vi "Copy of plot states.vi"() -> ()   [LabVIEW 2017]
panel:
  out "Ts Diagram":cluster{dbl[], dbl[]}[](graph)
  out "ph Diagram":cluster{dbl[], dbl[]}[](graph)
  out "Ts Sat Curve":cluster{dbl[], dbl[]}
  out "ph Sat Curve":cluster{dbl[], dbl[]}
  out "Ts output":cluster{dbl[], dbl[]}
  out "ph output":cluster{dbl[], dbl[]}
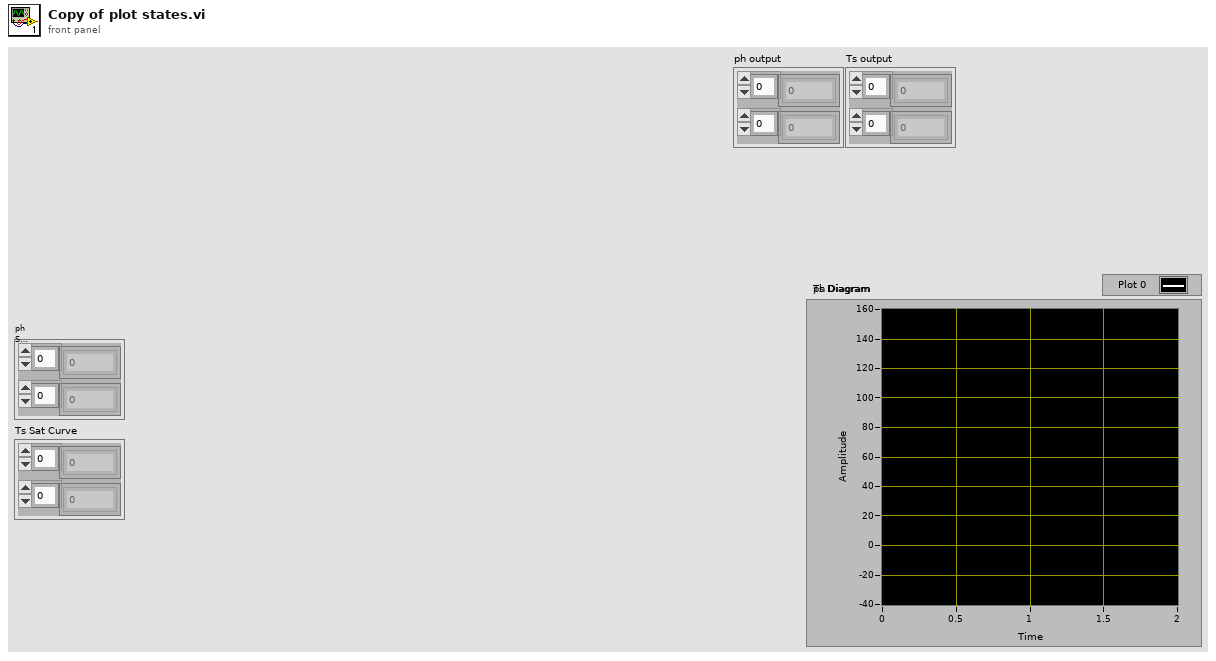
[diagram p1: front panel]
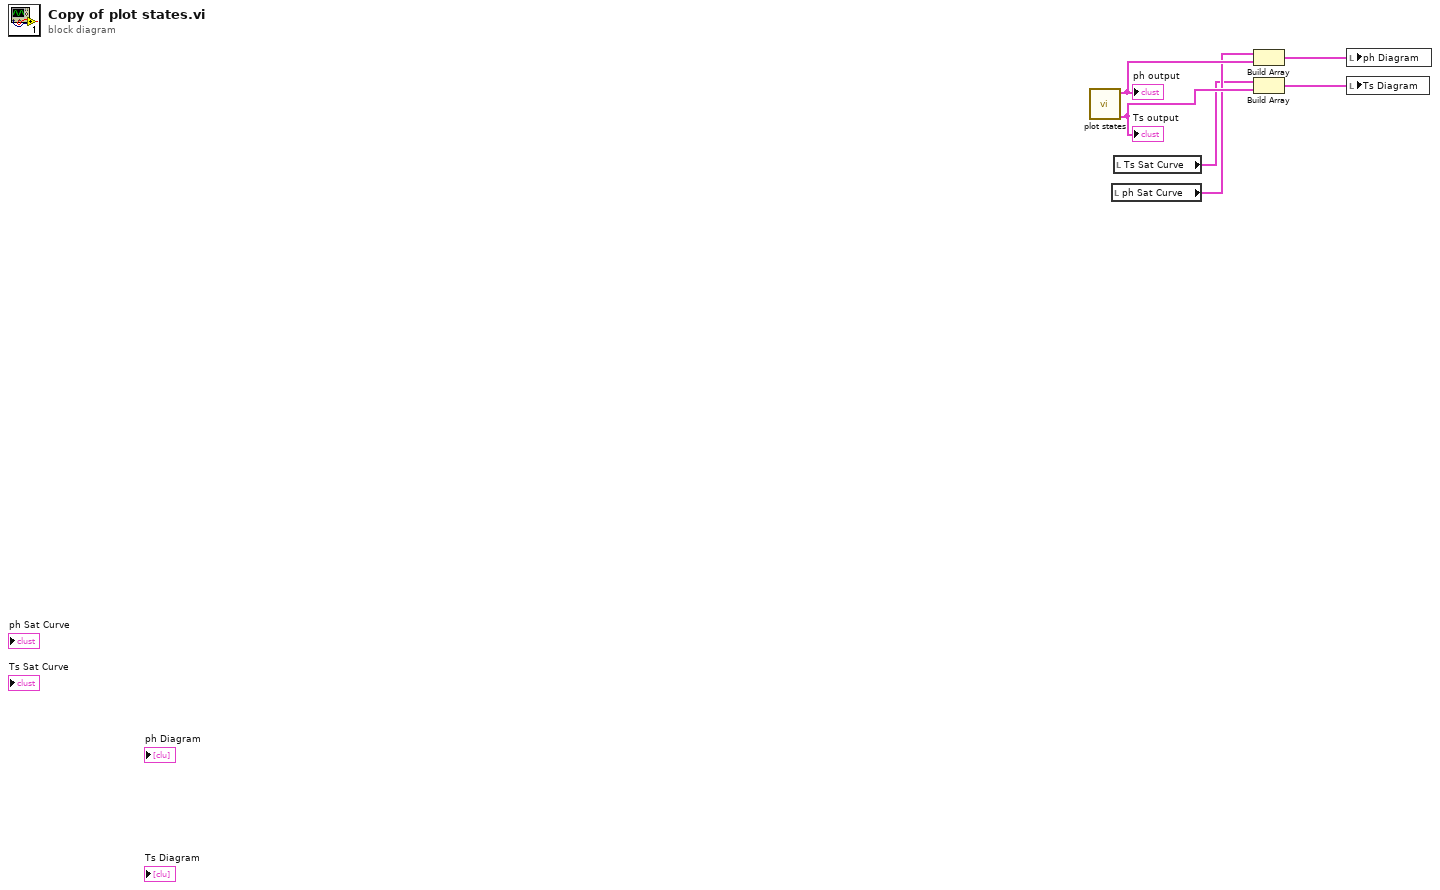
[diagram p0: block diagram]
diagram:
  n1 = call "plot states.vi"() -> ("Ts output"=w6:cluster{dbl[], dbl[]}, "ph output"=w5:cluster{dbl[], dbl[]})  [unwired: 10 in]
  "ph output" <- w5
  "Ts output" <- w6
  n2 = local read "ph Sat Curve"() -> (w4:cluster{dbl[], dbl[]})
  n3 = local read "Ts Sat Curve"() -> (w2:cluster{dbl[], dbl[]})
  n4 = Build Array(w4, w5) -> (w3:cluster{dbl[], dbl[]}[])
  n5 = Build Array(w2, w6) -> (w1:cluster{dbl[], dbl[]}[])
  n6 = local write "ph Diagram"(w3) -> ()
  n7 = local write "Ts Diagram"(w1) -> ()
